vi "File Wilt.vi"(0 "Dryer Aisle In":T1[](array[typedef]) {"Night Cycle Count" format="%04d"; "Dryer Details"."Stop Dryer" items=["NO", "YES"]; "Dryer Details"."24 Hour Water Injection" items=["NO", "YES"]; "Dryer Details"."Run w/o Newfi" items=["NO", "YES"]; "Day Cycle Count" format="%04d"}, 1 "Dryer Data Dir":path, 2 "RW  Mode":T3(ring), 5 "Dryer Bank Filename":path, 7 "Aisle Label":string="Aisle1", 9 "Last Save Hour":string="Aisle1", 11 "error in (no error)":errorcluster, 12 "Sample Data Current Filename":path) -> (4 "Dryer Aisle Out":T1[](array[typedef]) {"Night Cycle Count" format="%04d"; "Dryer Details"."Stop Dryer" items=["NO", "YES"]; "Dryer Details"."24 Hour Water Injection" items=["NO", "YES"]; "Dryer Details"."Run w/o Newfi" items=["NO", "YES"]; "Day Cycle Count" format="%04d"}, 6 "Last Save Hour Out":string, 8 "Sample Data Current Filename Out":path, 15 "error out":errorcluster)   [LabVIEW 2012]
uses:
  Dryer.ctl
  Dryer Details.ctl
  <vilib>/Utility/file.llb/Write To Spreadsheet File (string).vi
  <vilib>/Utility/file.llb/Read From Spreadsheet File (string).vi
panel:
  out "new file path (Not A Path if cancelled)":path
  out "first row":string[](array[string])
  out "mark after read (chars.)":i32
  out "all rows 2":string[][](array[string])
  in  "format (%s)":string="%s"
  in  "transpose (no:F)":bool
  in  "type (empty)":string[][](array[string])
  out "EOF?":bool
  out "all rows":string[][](array[string])
  # "D"
  # "N"
  # "D"
  # "N"
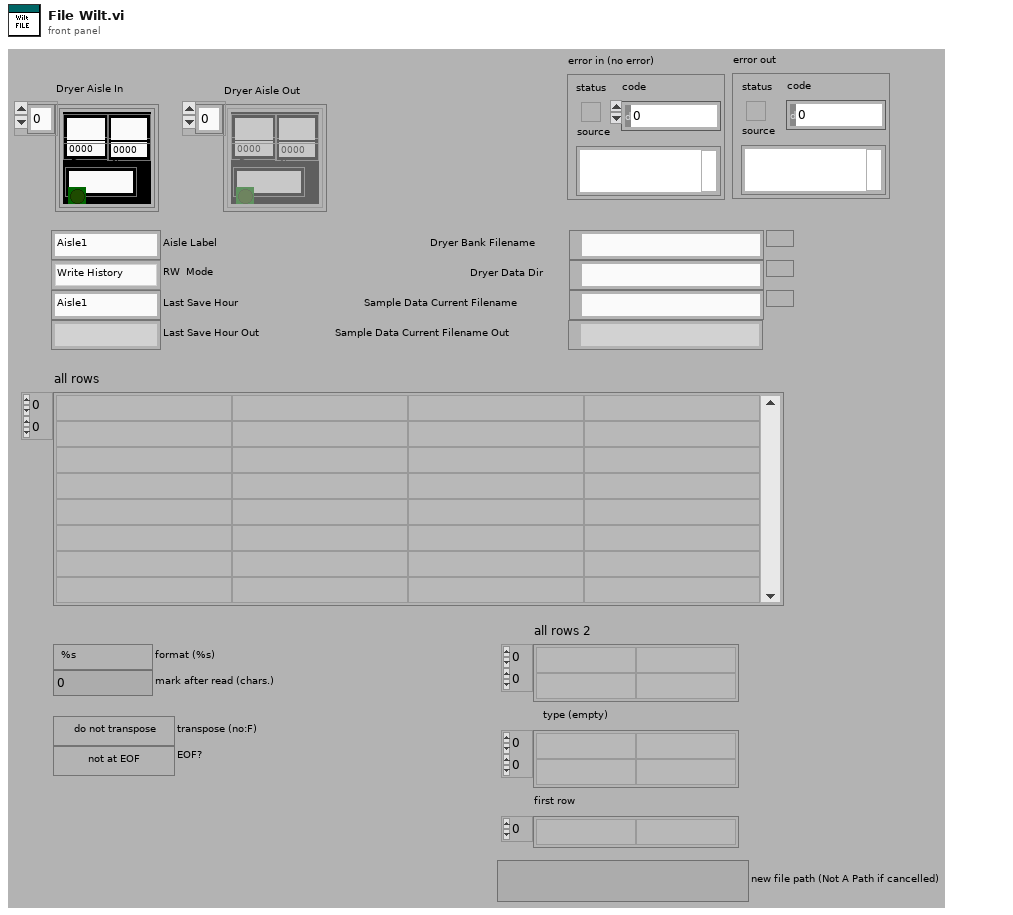
[diagram p1: front panel]
types:
  T1 = typedef "Dryer.ctl" = cluster{"Lab ID":string, "Day Cycle Count":i32, "Station Label":string, "Dryer Details":T2, "Sample Record ":string[], "Hist Record ":string[][], "Status Color":u32, "Boolean":bool, "Com Port":u8, "Bad Com Count":i32, "Current Run Start Time":dbl, "Night Cycle Count":i32, "Station Index":i32, "Cycle Index":string, "Audit Alert":bool}
  T2 = typedef "Dryer Details.ctl" = cluster{"Station":string, "Cycle Count Day":string, "Status":string, "Debug ASCII":string, "Notes":string, "Lab ID":string, "Total Time On":string, "TR Number":string, "Cycle Count Night":string, "Time On Day":string, "Time On Night":string, "Run w/o Newfi":i32, "24 Hour Water Injection":i32, "Stop Dryer":i32}
  T3 = enum16{"Write History", "Write Sample Data", "Write Dryer Bank", "Read Dryer Bank", "Read Sample History"}
  T4 = enum32{"Invalid", "Standard", "Closed", "Hidden", "Minimized", "Maximized"}
  T5 = enum16{"Read 2D Array", "Write 2D Array", "Write/Append 1D Array"}
  T6 = cluster{"This VI":refnum<vi>, "Dryer Aisle In":T1[], "Dryer Bank Filename":path, "Aisle Label":string, "Dryer Aisle Ot":T1[], "Dryer Data Dir":path, "Last Save Hour":string, "Sample Data Current Filename":path, "All Sample Data":string[][]}
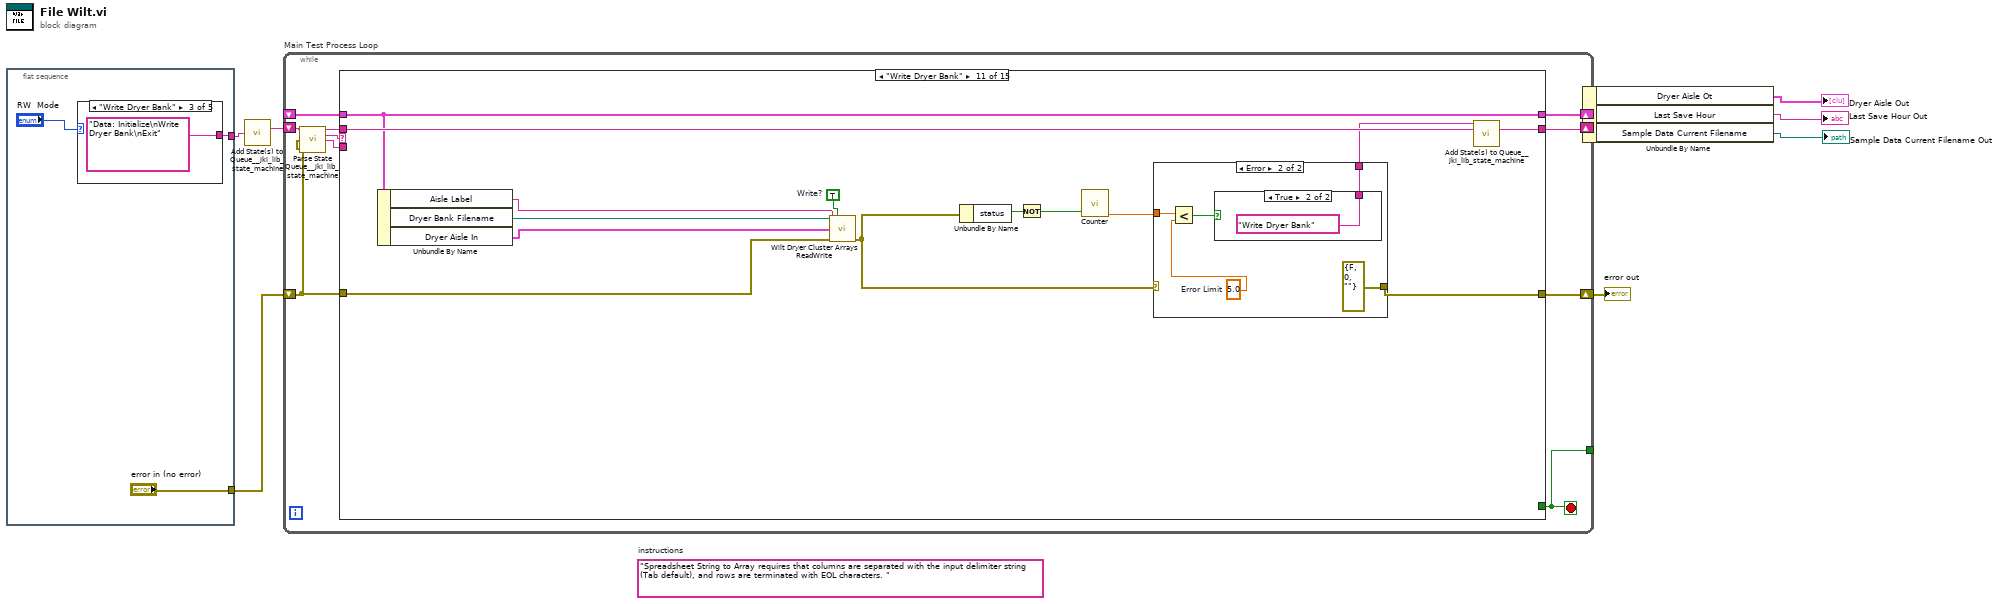
[diagram p0: block diagram]
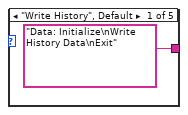
[diagram p2: hidden frame]
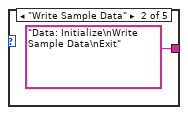
[diagram p3: hidden frame]
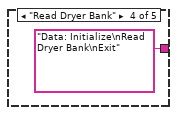
[diagram p4: hidden frame]
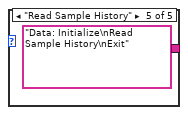
[diagram p5: hidden frame]
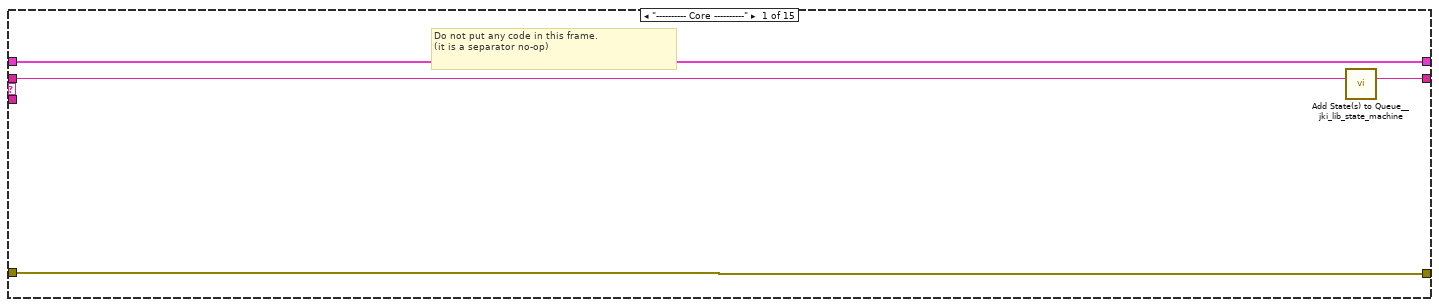
[diagram p6: hidden frame]
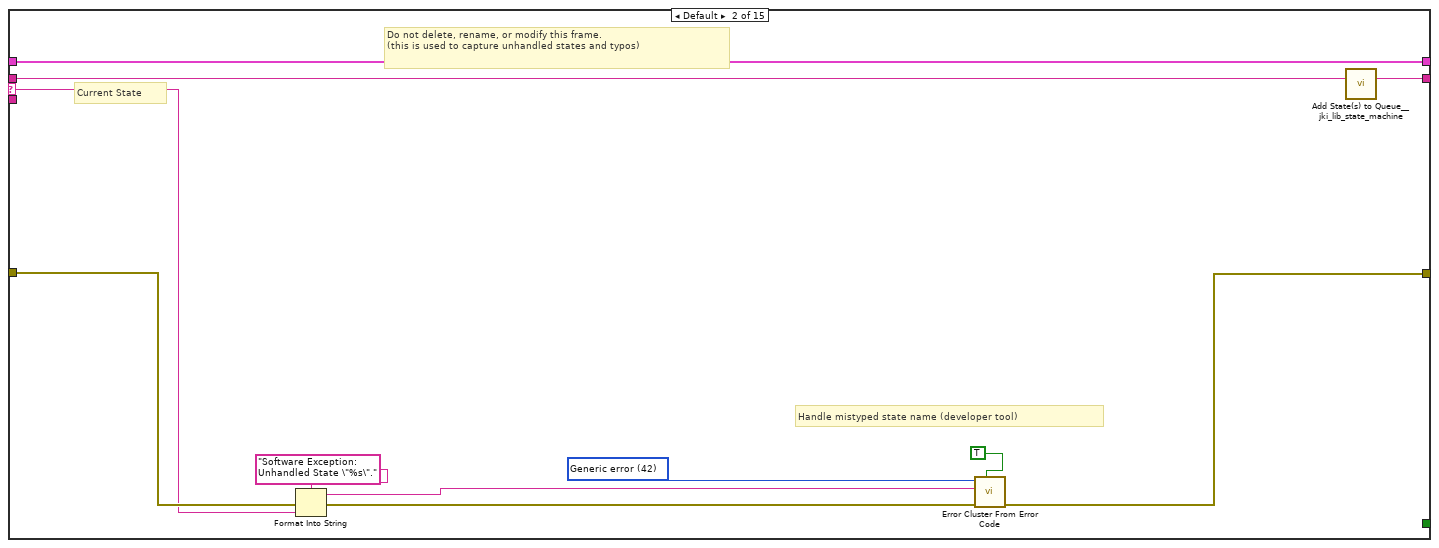
[diagram p7: hidden frame]
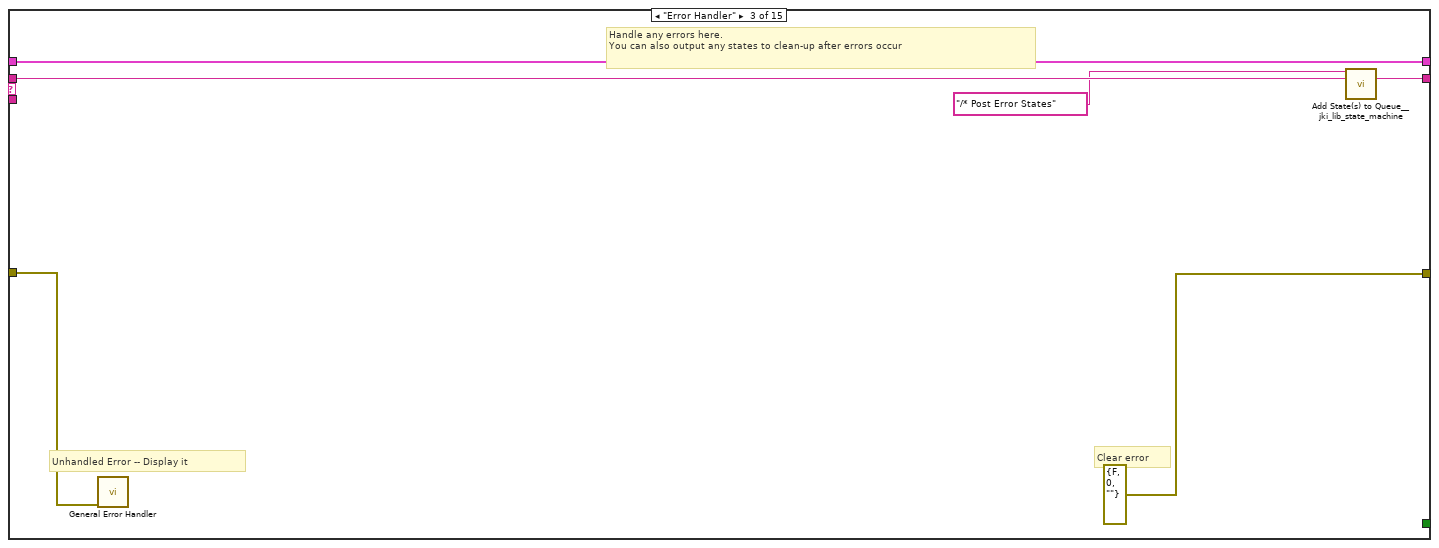
[diagram p8: hidden frame]
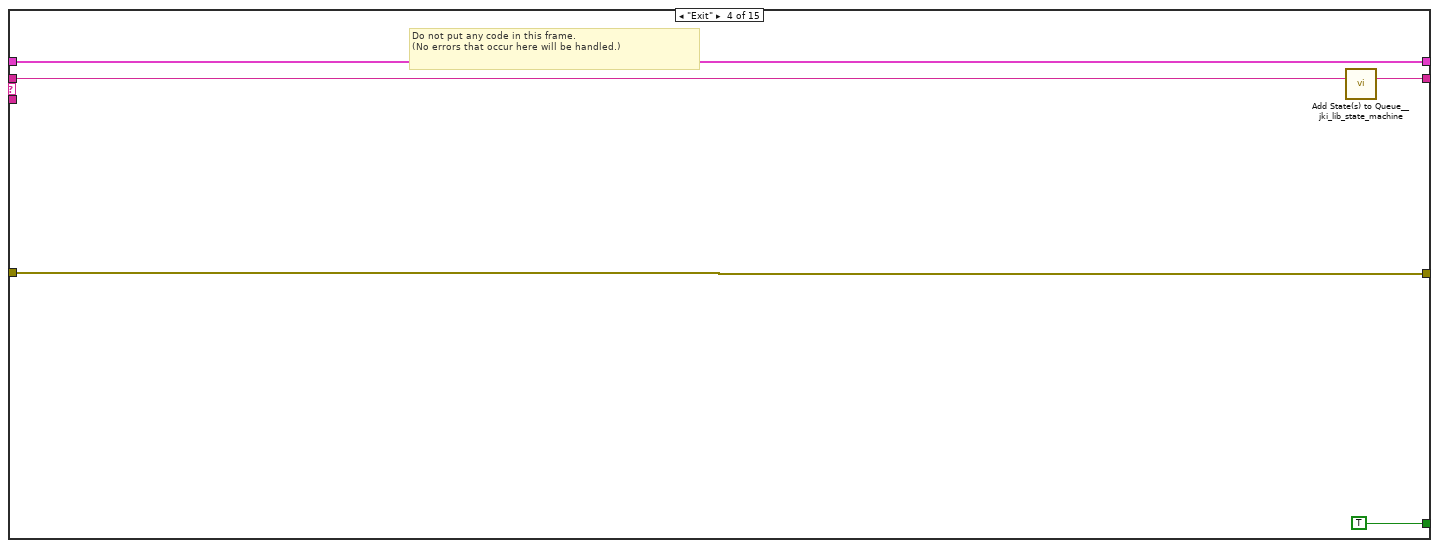
[diagram p9: hidden frame]
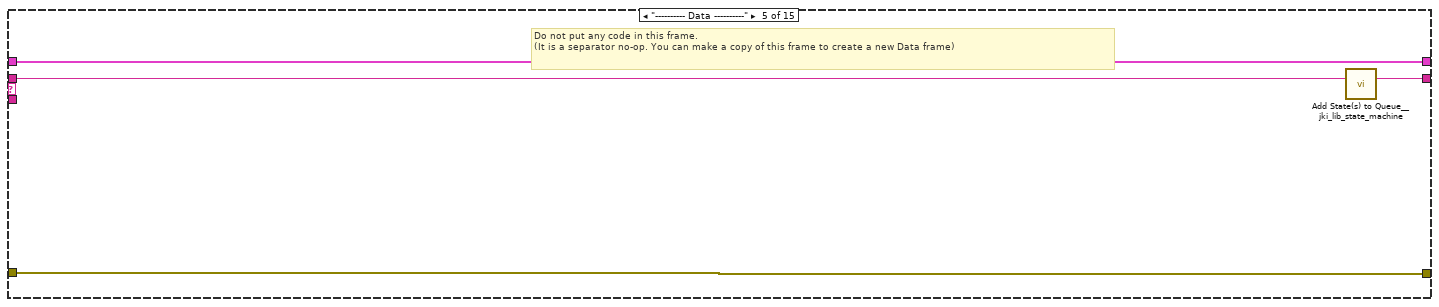
[diagram p10: hidden frame]
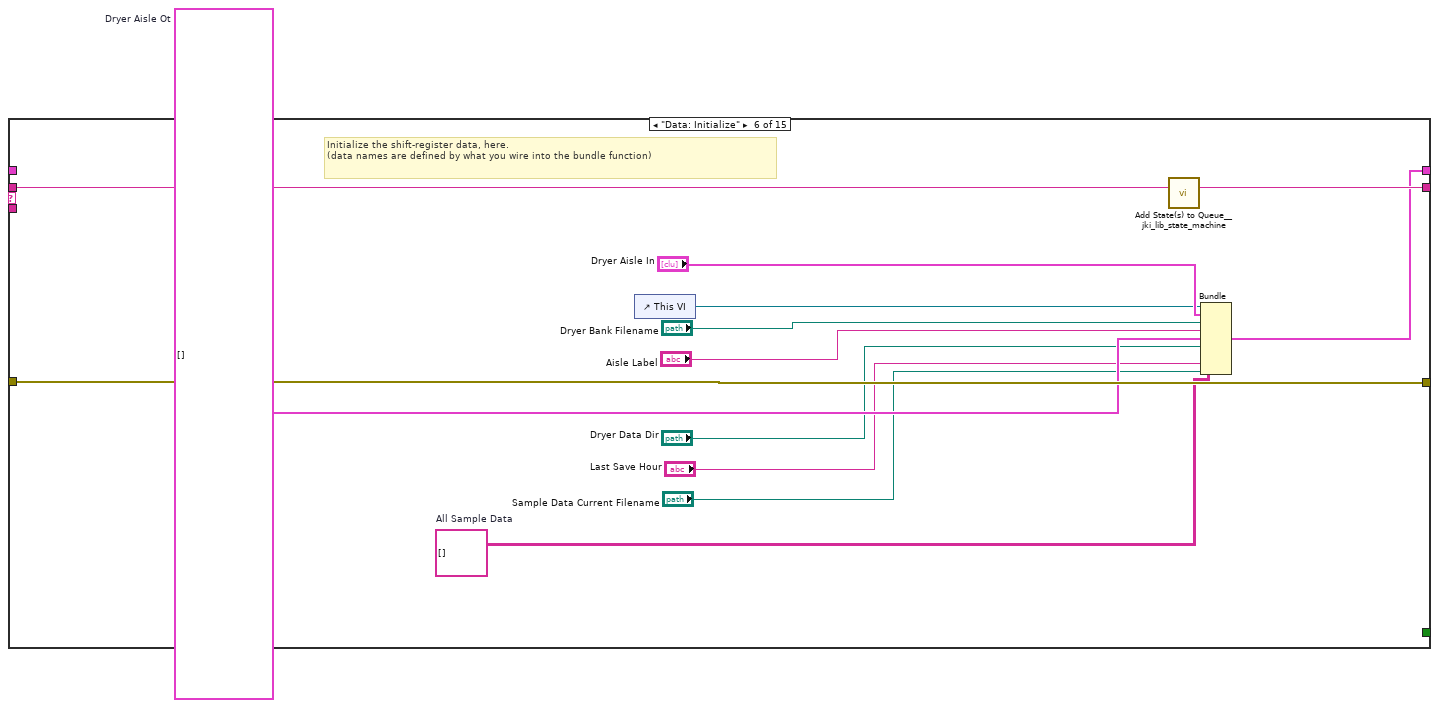
[diagram p11: hidden frame]
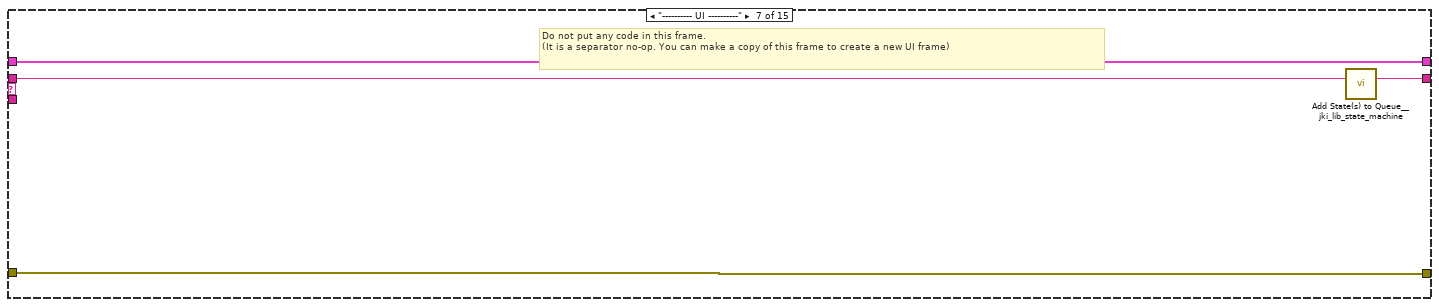
[diagram p12: hidden frame]
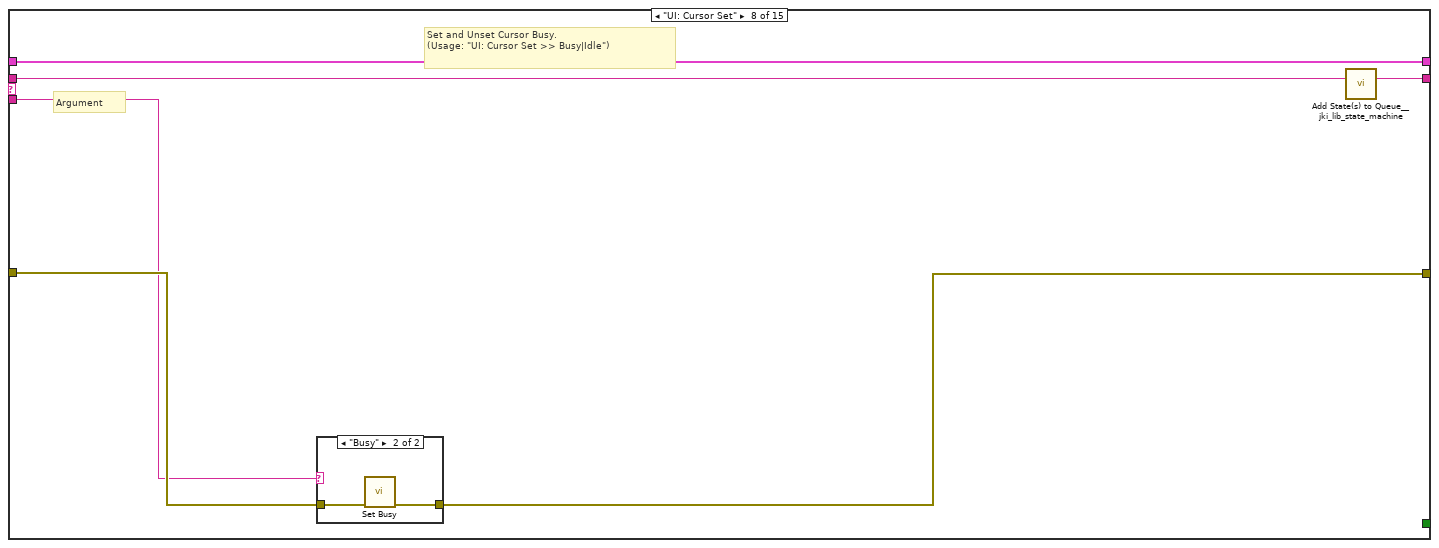
[diagram p13: hidden frame]
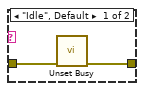
[diagram p14: hidden frame]
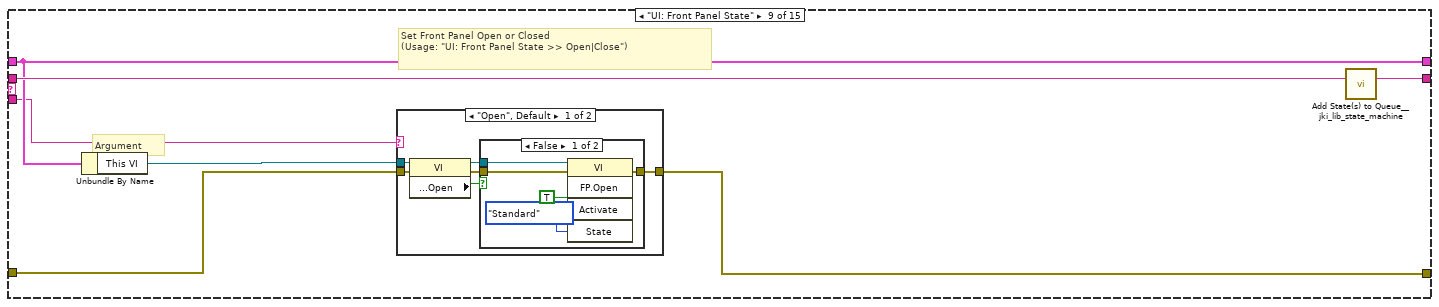
[diagram p15: hidden frame]
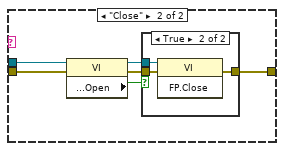
[diagram p17: hidden frame]
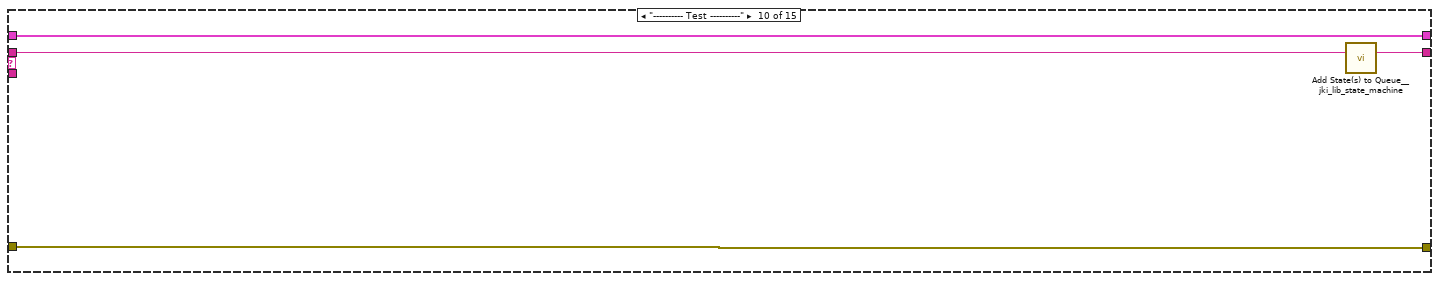
[diagram p19: hidden frame]
diagram:
  (unwired) "Spreadsheet String to Array requires that columns are separated with the input delimiter string (Tab default), and rows are terminated with EOL characters. "  # instructions
  n1 = flat-sequence {
    tunnel: [w11] -> w7
    tunnel: ["error in (no error)"] -> w3
    frame #0 {
      n2 = case shown="\"Write Dryer Bank\"" "RW  Mode" {
        tunnel: ["Data: Initialize\nWrite History Data\nExit" "Data: Initialize\nWrite Sample Data\nExit" "Data: Initialize\nWrite Dryer Bank\nExit" "Data: Initialize\nRead Dryer Bank\nExit" "Data: Initialize\nRead Sample History\nExit"] -> w11
        frame "Write History", Default {
        }
        frame "Write Sample Data" {
        }
        frame "Write Dryer Bank" {
        }
        frame "Read Dryer Bank" {
        }
        frame "Read Sample History" {
        }
      }
    }
  }
  n3 = call <vilib>:"Add State(s) to Queue__jki_lib_state_machine.vi"("State(s) at Back (\"\")"=w7) -> ("States Out"=w8:string)  [unwired: 14 in]
  n4 = while "Main Test Process Loop" {
    shift-right: [w20] -> w6
    shift-left: _ -> [w19]
    shift-right: [w22] -> w4
    shift-left: w3 -> [w18]
    shift-right: [w21] -> _
    shift-left: w8 -> [w23]
    tunnel: [w17] -> _
    stop <- w17 stop-if-true
    n5 = call <vilib>:"Parse State Queue__jki_lib_state_machine.vi"("State Queue"=w23, "Error In (no error)"=w18) -> ("Remaining States"=w25:string, "Current State"=w26:string, "Arguments"=w24:string)  [unwired: 11 in]
    n6 = case shown="\"Write Dryer Bank\"" w26 {
      selector: w26 -> [_ w31 _ _ _ _ _ _ _ _ _ _ _ _ _]
      tunnel: w25 -> [w30 w35 w47 w52 w56 w69 w73 w79 w90 w116 w130 w160 w179 w216 w239]
      tunnel: w24 -> [_ _ _ _ _ _ _ w74 w84 _ _ _ _ _ _]
      tunnel: w19 -> [w27 w33 w44 w50 w53 _ w70 w77 w86 w113 w128 w154 w177 w207 w237]
      tunnel: [w28 w37 errorcluster {"status"=FALSE, "code"=0, "source"=""} ("error out") w49 w54 w66 w71 w75 w87 w114 w117 w158 w174 w212 w234] -> w22
      tunnel: w18 -> [w28 w36 w43 w49 w54 w66 w71 w76 w88 w114 w125 w158 w174 w213 w234]
      tunnel: [w29 w34 w46 w51 w55 w68 w72 w78 w89 w115 w129 w159 w178 w215 w238] -> w21
      tunnel: [_ _ _ TRUE _ _ _ _ _ _ _ _ _ _ _] -> w17
      tunnel: [w27 w33 w44 w50 w53 w67 w70 w77 w86 w113 w128 w153 w177 w206 w236] -> w20
      frame "---------- Core ----------" {
        # "Do not put any code in this frame.\n(it is a separator no-op)"
        n7 = call <vilib>:"Add State(s) to Queue__jki_lib_state_machine.vi"("State(s) in (\"\")"=w30) -> ("States Out"=w29:string)  [unwired: 14 in]
      }
      frame Default {
        w40 = 42 items=["No error", "Argument error", "Memory is full", "Out of zone", "End of file", "File already open", "Generic file I/O error", "File not found", "File permission error", "Disk is full", "Duplicate path", "Too many files open", "System feature not enabled", "Resource file not found", "Cannot add resource", "Resource not found", "Image not found", "Image memory error", "Pen does not exist", "Config type invalid", "Config token not found", "Config parse error", "Config memory error", "Bad external code format", "Bad external code offset", "External code not present", "Null window", "Destroy window error", "Null menu", "Print aborted", "Bad print record", "Print driver error", "Windows error during printing", "Memory error during printing", "Print dialog error", "Generic print error", "Invalid device refnum", "Device not found", "Device parameter error", "Device unit error", "Cannot open device", "Device call aborted", "Generic error", "Cancelled by user", "Object ID too low", "Object ID too high", "Object not in heap", "Unknown heap", "Unknown object (invalid DefProc)", "Unknown object (DefProc not in table)", "Message out of range", "Invalid (null) method", "Unknown message", "Manager call not supported", "Bad address", "Network operation in progress", "Network operation timed out", "Connection is busy", "Network attribute not supported", "Network error", "Address in use", "System out of memory", "Connection aborted", "Connection refused", "Not connected", "Already connected", "Connection closed", "Initialization error (interapplication manager)", "Bad occurrence", "Wait on unbound occurrence handler", "Occurrence queue overflow", "Datalog type conflict", "Unused", "Unrecognized type (interapplication manager)", "Memory corrupt", "Failed to make temporary DLL", "Old CIN version", "Drag socket not found", "Failed to load drop-object", "Failed to register OLE object", "Failed to release OLE object", "Format specifier type mismatch", "Unknown format specifier", "Too few format specifiers", "Too many format specifiers", "Scan failed", "Newer CIN version", "Error converting to variant", "Runtime menu error", "Password tampered", "Variant attribute not found", "Incompatible variant data type", "Event data is not available", "Event Store is not present", "Occurrence is not found", "Event Queue is not created", "Event info is not available", "Refnum passed is NULL", "Error retrieving Class GUID", "Error retrieving CoClass GUID", "Error retrieving TypeLib GUID.", "Bad built application magic bytes.", "Specific driver is different from the specific driver associated with the Logical Name.", "There is no session opened to the class driver.", "Max Error", "MAX - Error with config objects", "MAX - Error loading configuration", "MAX - Group not supported"]
        # "Current State"
        # "Do not delete, rename, or modify this frame.\n(this is used to capture unhandled states and typos)"
        # "Handle mistyped state name (developer tool)"
        n8 = Format Into String(format string="Software Exception: Unhandled State \"%s\"." ("message"), error in=w36, w31) -> (resulting string=w39:string, error out=w38:errorcluster)  [unwired: 1 in]
        n9 = call <vilib>:"Error Cluster From Error Code.vi"("show call chain? (False)"=TRUE, "error in (no error)"=w38, "error message (\"\")"=w39, "error code (0)"=w40) -> ("error out"=w37:errorcluster)  [unwired: 5 in]
        n10 = call <vilib>:"Add State(s) to Queue__jki_lib_state_machine.vi"("State(s) in (\"\")"=w35) -> ("States Out"=w34:string)  [unwired: 14 in]
      }
      frame "Error Handler" {
        # "Unhandled Error -- Display it"
        # "Handle any errors here.\nYou can also output any states to clean-up after errors occur"
        # "Clear error"
        n11 = call <vilib>:"General Error Handler.vi"("error in (no error)"=w43) -> ()  [unwired: 10 in, 5 out]
        n12 = call <vilib>:"Add State(s) to Queue__jki_lib_state_machine.vi"("State(s) in Front (\"\")"="/* Post Error States", "State(s) in (\"\")"=w47) -> ("States Out"=w46:string)  [unwired: 13 in]
      }
      frame "Exit" {
        # "Do not put any code in this frame.\n(No errors that occur here will be handled.)"
        n13 = call <vilib>:"Add State(s) to Queue__jki_lib_state_machine.vi"("State(s) in (\"\")"=w52) -> ("States Out"=w51:string)  [unwired: 14 in]
      }
      frame "---------- Data ----------" {
        # "Do not put any code in this frame.\n(It is a separator no-op. You can make a copy of this frame to create a new Data frame)"
        n14 = call <vilib>:"Add State(s) to Queue__jki_lib_state_machine.vi"("State(s) in (\"\")"=w56) -> ("States Out"=w55:string)  [unwired: 14 in]
      }
      frame "Data: Initialize" {
        w57 = string[][] []  # All Sample Data
        w62 = T1[] []  # Dryer Aisle Ot
        # "Initialize the shift-register data, here.\n(data names are defined by what you wire into the bundle function)"
        n15 = control-ref of="This VI"() -> (w61:refnum<vi>)
        n16 = call <vilib>:"Add State(s) to Queue__jki_lib_state_machine.vi"("State(s) in (\"\")"=w69) -> ("States Out"=w68:string)  [unwired: 14 in]
        n17 = Bundle("This VI"=w61, "Dryer Aisle In"="Dryer Aisle In", "Dryer Bank Filename"="Dryer Bank Filename", "Aisle Label"="Aisle Label", "Dryer Aisle Ot"=w62, "Dryer Data Dir"="Dryer Data Dir", "Last Save Hour"="Last Save Hour", "Sample Data Current Filename"="Sample Data Current Filename", "All Sample Data"=w57) -> (w67:T6)  [unwired: 1 in]
      }
      frame "---------- UI ----------" {
        # "Do not put any code in this frame.\n(It is a separator no-op. You can make a copy of this frame to create a new UI frame)"
        n18 = call <vilib>:"Add State(s) to Queue__jki_lib_state_machine.vi"("State(s) in (\"\")"=w73) -> ("States Out"=w72:string)  [unwired: 14 in]
      }
      frame "UI: Cursor Set" {
        # "Argument"
        # "Set and Unset Cursor Busy.\n(Usage: \"UI: Cursor Set >> Busy|Idle\")"
        n19 = case shown="\"Busy\"" w74 {
          tunnel: w76 -> [w81 w83]
          tunnel: [w80 w82] -> w75
          frame "Idle", Default {
            n20 = call <vilib>:"Unset Busy.vi"("error in (no error)"=w81) -> ("error out"=w80:errorcluster)  [unwired: 10 in]
          }
          frame "Busy" {
            n21 = call <vilib>:"Set Busy.vi"("error in (no error)"=w83) -> ("error out"=w82:errorcluster)  [unwired: 9 in, 1 out]
          }
        }
        n22 = call <vilib>:"Add State(s) to Queue__jki_lib_state_machine.vi"("State(s) in (\"\")"=w79) -> ("States Out"=w78:string)  [unwired: 14 in]
      }
      frame "UI: Front Panel State" {
        # "Argument"
        # "Set Front Panel Open or Closed\n(Usage: \"UI: Front Panel State >> Open|Close\")"
        n23 = Unbundle By Name(w86) -> ("This VI"=w85:refnum<vi>)
        n24 = case shown="\"Open\", Default" w84 {
          tunnel: w88 -> [w94 w107]
          tunnel: [w96 w108] -> w87
          tunnel: w85 -> [w95 w105]
          frame "Open", Default {
            n25 = property class="VI"(reference=w95, error in=w94) -> (reference out=w92:refnum<vi>, error out=w93:errorcluster, "Front Panel.Open"=w91:bool)
            n26 = case shown="False" w91 {
              tunnel: [w99 w102] -> w96
              tunnel: w93 -> [w98 w102]
              tunnel: w92 -> [w97 _]
              frame False {
                n27 = invoke class="VI" method="FP.Open"(reference=w97, error in=w98, "Activate"=TRUE, "State"=T4."Standard") -> (error out=w99:errorcluster)  [unwired: 1 in, 4 out]
              }
              frame True {
              }
            }
          }
          frame "Close" {
            n28 = property class="VI"(reference=w105, error in=w107) -> (reference out=w104:refnum<vi>, error out=w106:errorcluster, "Front Panel.Open"=w103:bool)
            n29 = case shown="True" w103 {
              tunnel: [w109 w112] -> w108
              tunnel: w106 -> [w109 w111]
              tunnel: w104 -> [_ w110]
              frame False {
              }
              frame True {
                n30 = invoke class="VI" method="FP.Close"(reference=w110, error in=w111) -> (error out=w112:errorcluster)  [unwired: 1 in, 2 out]
              }
            }
          }
        }
        n31 = call <vilib>:"Add State(s) to Queue__jki_lib_state_machine.vi"("State(s) in (\"\")"=w90) -> ("States Out"=w89:string)  [unwired: 14 in]
      }
      frame "---------- Test ----------" {
        n32 = call <vilib>:"Add State(s) to Queue__jki_lib_state_machine.vi"("State(s) in (\"\")"=w116) -> ("States Out"=w115:string)  [unwired: 14 in]
      }
      frame "Write Dryer Bank" {
        w126 = TRUE  # Write?
        n33 = Unbundle By Name(w128) -> ("Aisle Label"=w123:string, "Dryer Bank Filename"=w124:path, "Dryer Aisle In"=w127:T1[])
        n34 = call "Wilt Dryer Cluster Arrays ReadWrite.vi"("Array Label"=w123, "Write?"=w126, "configuration file path"=w124, "Array Dryers In"=w127, "error in (no error)"=w125) -> ("error out"=w122:errorcluster)  [unwired: 9 in, 1 out]
        n35 = Unbundle By Name(w122) -> ("status"=w121:bool)
        n36 = Not(x=w121) -> (.not. x?=w120:bool)
        n37 = call "Counter.vi"("Reset"=w120) -> ("Count"=w119:dbl)  [unwired: 10 in]
        n38 = case shown="Error" w122 {
          selector: w122 -> [w131 _]
          tunnel: w119 -> [_ w136]
          tunnel: [_ w133] -> w118
          tunnel: [w131 errorcluster {"status"=FALSE, "code"=0, "source"=""} ("error IO")] -> w117
          frame No Error {
          }
          frame Error {
            w135 = 5.0  # Error Limit
            n39 = Less?(x=w136, y=w135) -> (x < y?=w134:bool)
            n40 = case shown="True" w134 {
              tunnel: [_ "Write Dryer Bank" ("State(s) in Front (\"\")")] -> w133
              frame False {
              }
              frame True {
              }
            }
          }
        }
        n41 = call <vilib>:"Add State(s) to Queue__jki_lib_state_machine.vi"("State(s) in Front (\"\")"=w118, "State(s) in (\"\")"=w130) -> ("States Out"=w129:string)  [unwired: 13 in]
      }
      frame "Write Sample Data" {
        # "New Hour"
        n42 = Unbundle By Name(w154) -> ("Dryer Data Dir"=w143:path, "Sample Data Current Filename"=w144:path, "Dryer Aisle In"=w157:T1[], "Last Save Hour"=w156:string)
        n43 = Format Date/Time String(time format string (%c)="%H") -> (date/time string=w152:string)  [unwired: 2 out]
        n44 = Not Equal?(x=w156, y=w152) -> (x != y?=w151:bool)
        n45 = for {
          tunnel: w157 -> [w173] mode=indexing
          shift-right: [w171] -> w148
          shift-left: string[] [] -> [w169]
          # "Fix ASCII replaces multiline feedback with other delimiters."
          n46 = Unbundle By Name(w173) -> ("Sample Record"=w166:string[])
          n47 = call "Sample Array - Fix Ascii.vi"("Sample Array In"=w166) -> ("Sample Array Out"=w167:string[])  [unwired: 10 in]
          n48 = Replace Array Subset(array=string[] ["t", "CC", "Tc", "ASCII", "STATUS", "L1", "L2", "trmb", "v", "v2", "sw"], new element=w167, index=0 ("index (row)")) -> (w168:string[])
          n49 = Build Array (concatenate)(w169, w168) -> (w171:string[])
        }
        n50 = call "Counter.vi"() -> ("Count"=w150:dbl)  [unwired: 11 in]
        n51 = To Unsigned Long Integer(number=w150) -> (unsigned 32bit integer=w141:u32)
        n52 = Number To Decimal String(number=w141) -> (decimal integer string=w139:string)  [unwired: 1 in]
        n53 = Format Date/Time String(time format string (%c)="%m/%d/%Y - %H:%M:%S - ") -> (date/time string=w140:string)  [unwired: 2 out]
        n54 = Concatenate Strings(w140, w139) -> (w138:string)
        n55 = Build Array (concatenate)(w138, w148) -> (w146:string[])
        n56 = case shown="True" w151 {
          tunnel: w157 -> [_ w165]
          tunnel: w143 -> [_ w164]
          tunnel: [w161 w162] -> w147
          tunnel: w144 -> [w161 _]
          frame False {
          }
          frame True {
            n57 = call "File Create Wilt.vi"("base path"=w164, "File Record Type"=enum16{"History", "Sample", "Big Sample", ""}."Big Sample", "All Dryer Array In"=w165) -> ("appended path"=w162:path)  [unwired: 12 in]
          }
        }
        n58 = local write "Sample Data Current Filename"(w147) -> ()
        n59 = Bundle By Name(cluster=w154, "Last Save Hour"=w152, "Sample Data Current Filename"=w147) -> (w153:T6)
        n60 = call "Array 2D RW str.vi"("file path (dialog if empty)"=w147, "Write/Read"=T5."Write/Append 1D Array", "1D Sample Append Array"=w146) -> ()  [unwired: 12 in, 1 out]
        n61 = call <vilib>:"Add State(s) to Queue__jki_lib_state_machine.vi"("State(s) in (\"\")"=w160) -> ("States Out"=w159:string)  [unwired: 14 in]
      }
      frame "Write History Data" {
        n62 = Unbundle By Name(w177) -> ("Dryer Data Dir"=w175:path, "Dryer Aisle In"=w176:T1[])
        n63 = for {
          tunnel: w176 -> [w191] mode=indexing
          tunnel: w175 -> [w192]
          # "First sample, write to history file."
          n64 = Unbundle By Name(w191) -> ("Lab ID"=w188:string, "Station Label"=w180:string, "Dryer Details.Status"=w187:string)
          n65 = Unbundle By Name(w191) -> ("Hist Record"=w182:string[][])
          n66 = Build Array(w188, w180, w187) -> (w184:string[])
          n67 = Replace Array Subset(array=string[][] [["Serial Number", ""], ["Station", ""], ["Status", " "]] ("Hist Record(Cycle Count, t-comp,L1max, L2max, Tmax)"), new element=w184, index (col)=1 ("disabled index (col)")) -> (w183:string[][])  [unwired: 1 in]
          n68 = Build Array (concatenate)(w183, w182) -> (w181:string[][])
          n69 = call <vilib>:"Check if File or Folder Exists.vi"("path"=w192) -> ("file or folder exists?"=w190:bool, "dup path"=w189:path)  [unwired: 8 in, 1 out]
          n70 = case shown="False" w190 {
            tunnel: w181 -> [w193 w198]
            tunnel: w192 -> [_ w205]
            tunnel: w191 -> [_ w204]
            tunnel: w189 -> [w194 _]
            frame True {
              n71 = call-poly <vilib>:"Write To Spreadsheet File.vi"("delimiter (\\t)"="," ("delimiter (\\t)"), "append to file? (new file:F)"=TRUE, "2D data"=w193, "file path (dialog if empty)"=w194) -> ()  [unwired: 4 in, 1 out]
            }
            frame False {
              n72 = call "File Create Wilt.vi"("base path"=w205, "File Record Type"=enum16{"History", "Sample", "Big Sample", ""}."History", "Single Dryer In"=w204) -> ("appended path"=w199:path)  [unwired: 12 in]
              n73 = Index Array(array=w198, index (row)=0) -> (element=w200:string[])  [unwired: 1 in]
              n74 = call-poly <vilib>:"Write To Spreadsheet File.vi"("delimiter (\\t)"="," ("delimiter (\\t)"), "append to file? (new file:F)"=TRUE, "1D data"=w200, "file path (dialog if empty)"=w199) -> ()  [unwired: 4 in, 1 out]
            }
          }
        }
        n75 = call <vilib>:"Add State(s) to Queue__jki_lib_state_machine.vi"("State(s) in (\"\")"=w179) -> ("States Out"=w178:string)  [unwired: 14 in]
      }
      frame "Read Dryer Bank" {
        w214 = FALSE  # Write?
        n76 = Unbundle By Name(w207) -> ("Aisle Label"=w210:string, "Dryer Bank Filename"=w211:path, "Dryer Aisle In"=w209:T1[])
        n77 = call "Wilt Dryer Cluster Arrays ReadWrite.vi"("Array Label"=w210, "Write?"=w214, "configuration file path"=w211, "Array Dryers In"=w209, "error in (no error)"=w213) -> ("Array Dryers Out"=w208:T1[], "error out"=w212:errorcluster)  [unwired: 9 in]
        n78 = Bundle By Name(cluster=w207, "Dryer Aisle Ot"=w208) -> (w206:T6)
        n79 = call <vilib>:"Add State(s) to Queue__jki_lib_state_machine.vi"("State(s) in (\"\")"=w216) -> ("States Out"=w215:string)  [unwired: 14 in]
      }
      frame "Read Sample History" {
        w220 = 0  # max characters/row  (no limit:0)
        w221 = 0  # start of read offset (chars.:0)
        w219 = -1  # number of rows (all:-1)
        n80 = Unbundle By Name(w237) -> ("Sample Data Current Filename"=w217:path)
        n81 = call-poly <vilib>:"Read From Spreadsheet File.vi"("delimiter (\\t)"="," ("delimiter (\\t)"), "file path (dialog if empty)"=w217) -> ("all rows"=w233:string[][])  [unwired: 5 in, 4 out]
        "all rows" <- w233
        n82 = call <vilib>:"Read Lines From File.vi"("file path (dialog if empty)"=w217, "number of lines (all:-1)"=w219, "start of read offset (chars.:0)"=w221, "[max characters per line]  (no limit:0)"=w220) -> ("new file path (Not A Path if cancelled)"=→"new file path (Not A Path if cancelled)":path, "line string"=w222:string, "mark after read (chars.)"=→"mark after read (chars.)":i32, "EOF?"=→"EOF?":bool)  [unwired: 2 in]
        n83 = Spreadsheet String To Array(delimiter (Tab)="," ("delimiter (\\t)"), format string="format (%s)", spreadsheet string=w222, array type (2D Dbl)="type (empty)") -> (array=w230:string[][])
        n84 = case shown="True" "transpose (no:F)" {
          tunnel: w230 -> [w240 w242]
          tunnel: [w240 w241] -> w232
          frame False {
          }
          frame True {
            n85 = Transpose 2D Array(2D array=w242) -> (transposed array=w241:string[][])
          }
        }
        "all rows 2" <- w232
        n86 = Bundle By Name(cluster=w237, "All Sample Data"=w233) -> (w236:T6)
        n87 = Index Array(array=w232, index (row)=0) -> (element=→"first row":string[])  [unwired: 1 in]
        n88 = call <vilib>:"Add State(s) to Queue__jki_lib_state_machine.vi"("State(s) in (\"\")"=w239) -> ("States Out"=w238:string)  [unwired: 14 in]
      }
    }
  }
  "error out" <- w4
  n89 = Unbundle By Name(w6) -> ("Dryer Aisle Ot"=→"Dryer Aisle Out":T1[], "Last Save Hour"=→"Last Save Hour Out":string, "Sample Data Current Filename"=→"Sample Data Current Filename Out":path)
